vi "nPoints Concept - Hall Effect.vi"() -> ()   [LabVIEW 2014]
uses:
  <vilib>/DAQmx/create/channels.llb/DAQmx Create Channel (AI-Voltage-Basic).vi
  <vilib>/DAQmx/read.llb/DAQmx Read (Analog DBL 1Chan 1Samp).vi
panel:
  in  "Animation Settings":T1={"Number of Particles"=12, "px/s"=150, "Origin"={"X"=300, "Y"=150}, "Jitter"=1.0, "Seperation"=34, "X Max"=410}
  out "Meter":dbl(knob) scale=0.0..5.0
  out "Gravity":dbl(slide)=10.0 scale=-1.0..1.0
  out "new picture":picture
  in  "milliseconds to wait":u32=50
  out "Waveform Chart":dbl(graph)
  in  "Stop Button":bool
  # "Hall Effect Sensor"
  # "+5V"
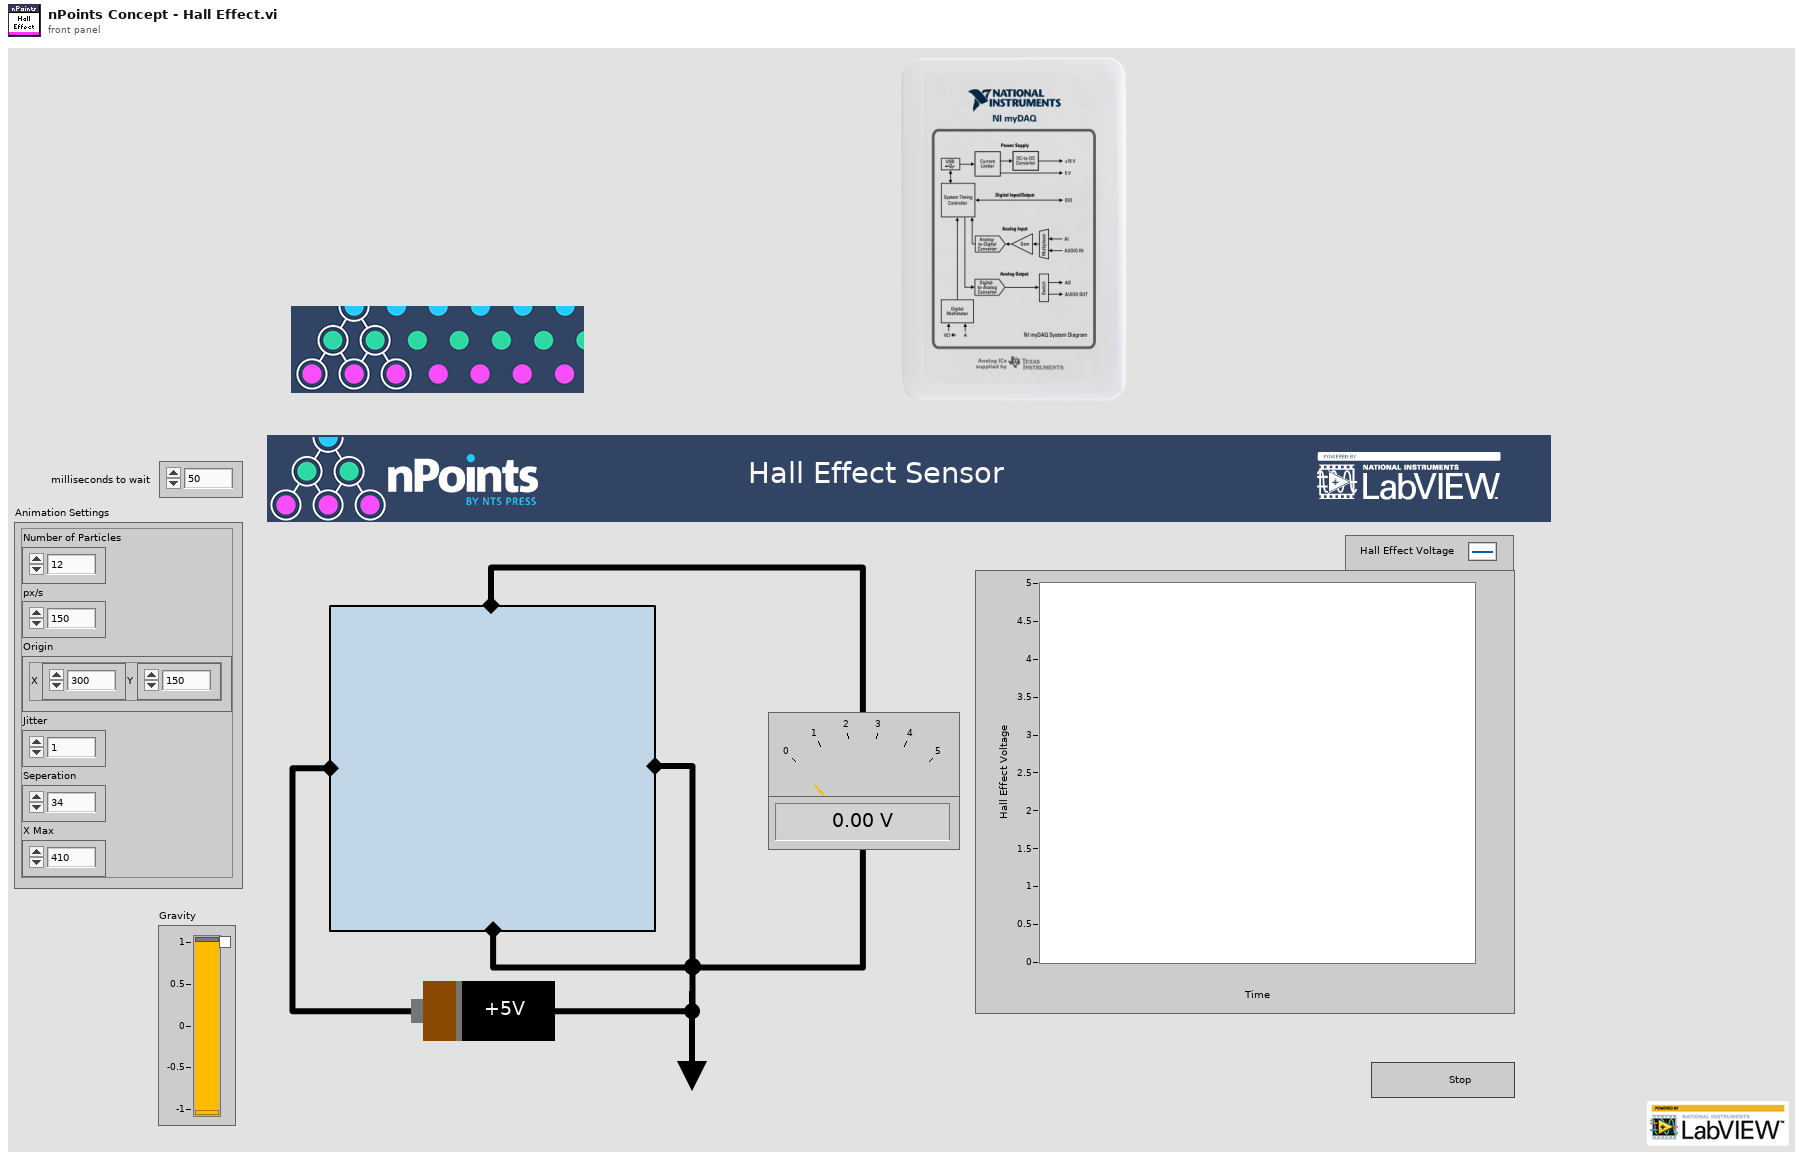
[diagram p1: front panel]
types:
  T1 = cluster{"Number of Particles":u32, "px/s":i32, "Origin":cluster{"X":i32, "Y":i32}, "Jitter":dbl, "Seperation":i32, "X Max":i32}
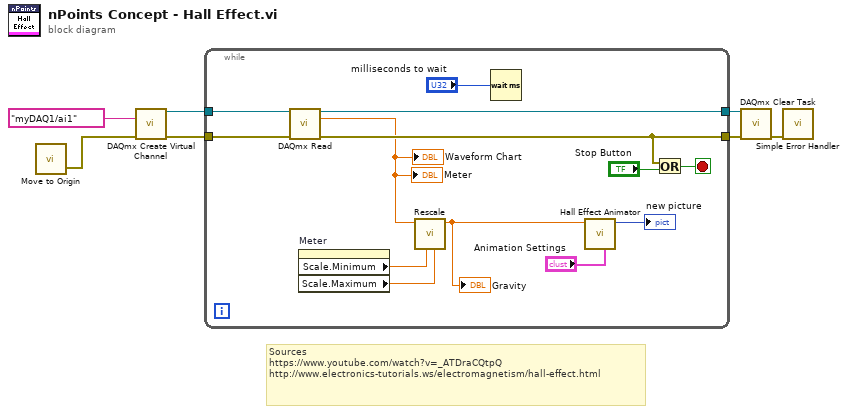
[diagram p0: block diagram]
diagram:
  # "Sources\nhttps://www.youtube.com/watch?v=_ATDraCQtpQ\nhttp://www.electronics-tutorials.ws/electromagnetism/hall-effect.html"
  n1 = call "Move to Origin.vi"() -> ("Error Out"=w1:errorcluster)  [unwired: 3 in]
  n2 = call-poly <vilib>:"DAQmx Create Virtual Channel.vi"("physical channels"=tag "myDAQ1/ai1", "error in"=w1) -> ("task out"=w6:refnum<k21>, "error out"=w5:errorcluster)  [unwired: 12 in]
  n3 = while {
    tunnel: w6 -> [w20]
    tunnel: w5 -> [w19]
    tunnel: [w18] -> w3
    tunnel: [w17] -> w2
    stop <- w15 stop-if-true
    n4 = call-poly <vilib>:"DAQmx Read.vi"("task/channels in"=w20, "error in"=w19) -> ("task out"=w17:refnum<k21>, "data"=w14:dbl, "error out"=w18:errorcluster)  [unwired: 11 in]
    "Waveform Chart" <- w14
    "Meter" <- w14
    n5 = property on="Meter" class="Knob (strict)"() -> ("Scale.Minimum"=w9:dbl, "Scale.Maximum"=w13:dbl)  [unwired: 2 in, 2 out]
    n6 = call "Rescale.vi"("Max In"=w13, "Min In"=w9, "Input"=w14) -> ("Output"=w11:dbl)  [unwired: 8 in]
    "Gravity" <- w11
    n7 = Wait (ms)(milliseconds to wait="milliseconds to wait") -> ()  [unwired: 1 out]
    n8 = call "Hall Effect Animator.vi"("Animation Settings"="Animation Settings", "Gravity"=w11) -> ("new picture"=→"new picture":picture)  [unwired: 8 in, 1 out]
    n9 = Or(x=w18, y="Stop Button") -> (x .or. y?=w15:bool)
  }
  n10 = call <vilib>:"DAQmx Clear Task.vi"("task in"=w2, "error in"=w3) -> ("error out"=w4:errorcluster)  [unwired: 13 in]
  n11 = call <vilib>:"Simple Error Handler.vi"("error in (no error)"=w4) -> ()  [unwired: 4 in, 5 out]
